vi "Write Gantry Region.vi"(8 "error in (no error)":errorcluster, 10 "Gantry Region":i32, 11 "Fixture in":refnum<class "Fixture.lvclass">) -> (0 "error out":errorcluster, 3 "Fixture out":refnum<class "Fixture.lvclass">)   [LabVIEW 2019, in "Fixture.lvclass"]
uses:
  Fixture.lvclass
  Fixture.lvclass/Fixture.ctl
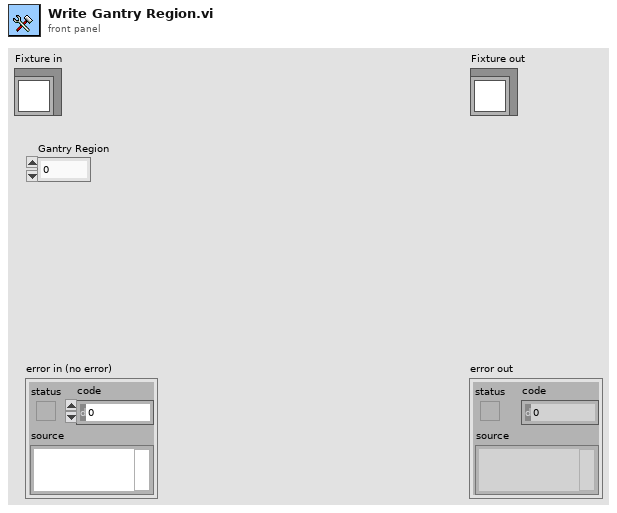
[diagram p1: front panel]
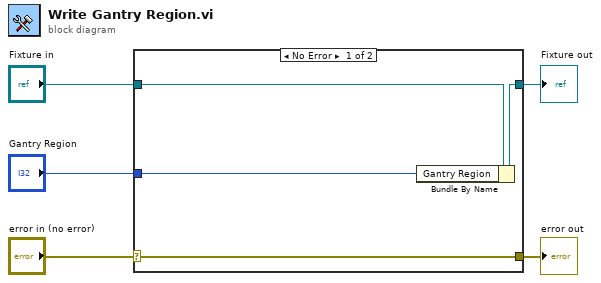
[diagram p0: block diagram]
diagram:
  n1 = case shown="No Error" "error in (no error)" {
    selector: "error in (no error)" -> [w9 w10]
    tunnel: [w9 w10] -> w4
    tunnel: [w7 w11] -> w2
    tunnel: "Fixture in" -> [w8 w11]
    tunnel: "Gantry Region" -> [w6 _]
    frame No Error {
      n2 = Bundle By Name(cluster=w8, "Gantry Region"=w6) -> (w7:refnum<class "Fixture.lvclass">)
    }
    frame Error {
    }
  }
  "error out" <- w4
  "Fixture out" <- w2
